vi "PS35_MotorInit.vi"(2 "error in (no error)":errorcluster, 3 "Axis number":i32=1 min=1 max=3, 4 "Control unit ID":i32=1 min=1 max=10) -> (0 "error out":errorcluster)   [LabVIEW 2020]
doc: "PS35_MotorInit.vi, created: 04.03.2009 alex; last change: 22.10.2019 alex;\n\n<B>FUNCTION:</B> \n\nInitialize an axis and switch on.\nWith this function the axis is completely initialized and afterwards is \nwith a current and with active positioning regulator.\nIt must be executed after the turning on of the control unit, so that the\naxis can be moved afterwards with the commands REF, PGO, VGO etc.\nBefore the following parameters must have been set: limit switch mask\nand polarity, start regulator parameters.\n----------------------------------------------------------------------------------------\n<B>INPUT:</B>\n[I32] <B>Control unit ID:</B> control unit index. (Default=1, Range=1...10) \n[I32] <B>Axis number:</B> axis number. (Default=1, Range=1...3) \n[CLU] <B>error in</B>\n----------------------------------------------------------------------------------------\n<B>OUTPUT:</B>\n[CLU] <B>error out</B>\n----------------------------------------------------------------------------------------\n<B>SUB-VIs:</B>\n----------------------------------------------------------------------------------------\n<B>EXT-Calls:</B>\nps35.dll (V2.01)\n----------------------------------------------------------------------------------------"
uses:
  ps35.dll
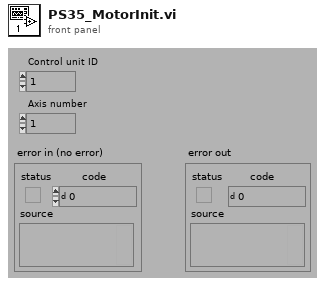
[diagram p1: front panel]
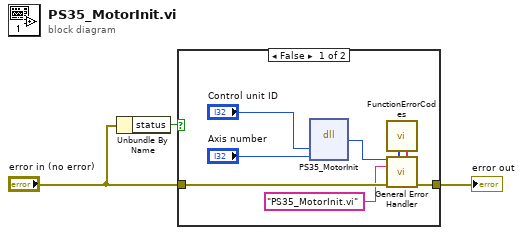
[diagram p0: block diagram]
diagram:
  n1 = Unbundle By Name("error in (no error)") -> ("status"=w1:bool)
  n2 = case shown="False" w1 {
    tunnel: "error in (no error)" -> [w10 w12]
    tunnel: [w9 w12] -> w3
    frame False {
      n3 = dll-call lib="C:/GEECS/Developers Version/source/Device Drivers/OwiSoft/OWISoftOEM/ps35/labview/lv82/ps35.dll" fn="PS35_MotorInit"("Index"="Control unit ID", "AxisNr"="Axis number") -> ("Rückgabetyp"=w8:i32)  [unwired: 5 in, 2 out]
      n4 = call "FunctionErrorCodes.vi"() -> ("[user-defined codes]"=w5:i32[], "[user-defined descriptions]"=w4:string[])  [unwired: 8 in]
      n5 = call <vilib>:"General Error Handler.vi"("[error code] (0)"=w8, "[user-defined codes]"=w5, "[user-defined descriptions]"=w4, "[error source] (\" \")"="PS35_MotorInit.vi" ("[error source] (\" \")"), "error in (no error)"=w10) -> ("error out"=w9:errorcluster)  [unwired: 6 in, 4 out]
    }
    frame True {
    }
  }
  "error out" <- w3
